vi "Add Custom Device Channel - Offline.vi"(4 "Property Values":variant[](array[variant]), 5 "Highlight? (F)":bool, 6 "Property names":string[](array[string]), 7 "GUID (Default Channel)":string="03D3BB99-1485-13A6-561D1F898F032919", 8 "error in (no error)":errorcluster, 9 "Channel":T2, 10 "Channel Name":string, 11 "Parent Ref in":T1 format="%.0x") -> (0 "error out":errorcluster, 1 "Channel Ref":T1 format="%.0x", 2 "Newly Created?":bool, 3 "Parent Ref out":T1 format="%.0x")   [LabVIEW 2017, in "Scan Engine Custom Device.lvlib"]
uses:
  Scan Engine Custom Device.lvlib
  <vilib>/NI Veristand/Custom Device API/Custom Device Item Ref.ctl
  <vilib>/NI Veristand/Custom Device API/Custom Device Channel.ctl
  <vilib>/NI Veristand/Custom Device API/Custom Device Channel Type.ctl
  NationalInstruments.VeriStand.SystemDefinitionAPI
  <vilib>/NI Veristand/Custom Device Offline API/Custom Device Offline API.lvlib
  <vilib>/NI Veristand/Custom Device API/Custom Device API.lvlib
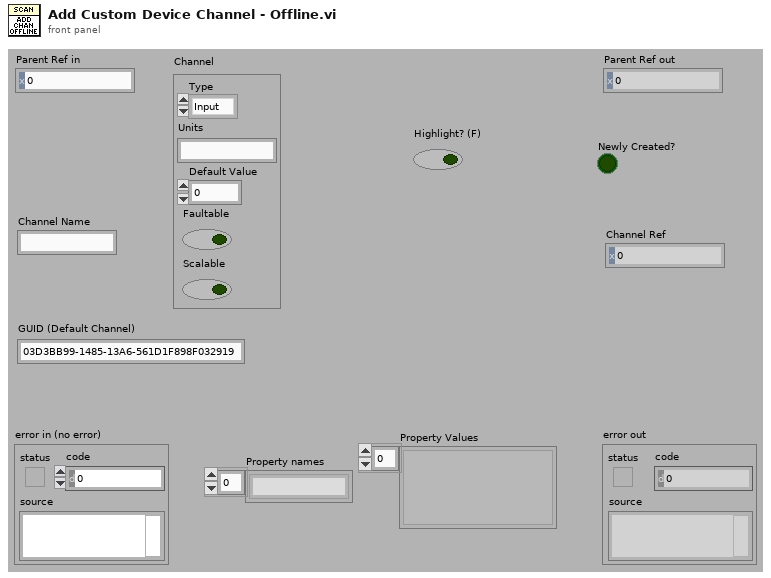
[diagram p1: front panel]
types:
  T1 = typedef "Custom Device API.lvlib/Custom Device Item Ref.ctl" = u64
  T2 = typedef "Custom Device API.lvlib/Custom Device Channel.ctl" = cluster{"Type":T3, "Units":string, "Default Value":dbl, "Faultable":bool, "Scalable":bool}
  T3 = typedef "Custom Device API.lvlib/Custom Device Channel Type.ctl" = enum16{"Input", "Output"}
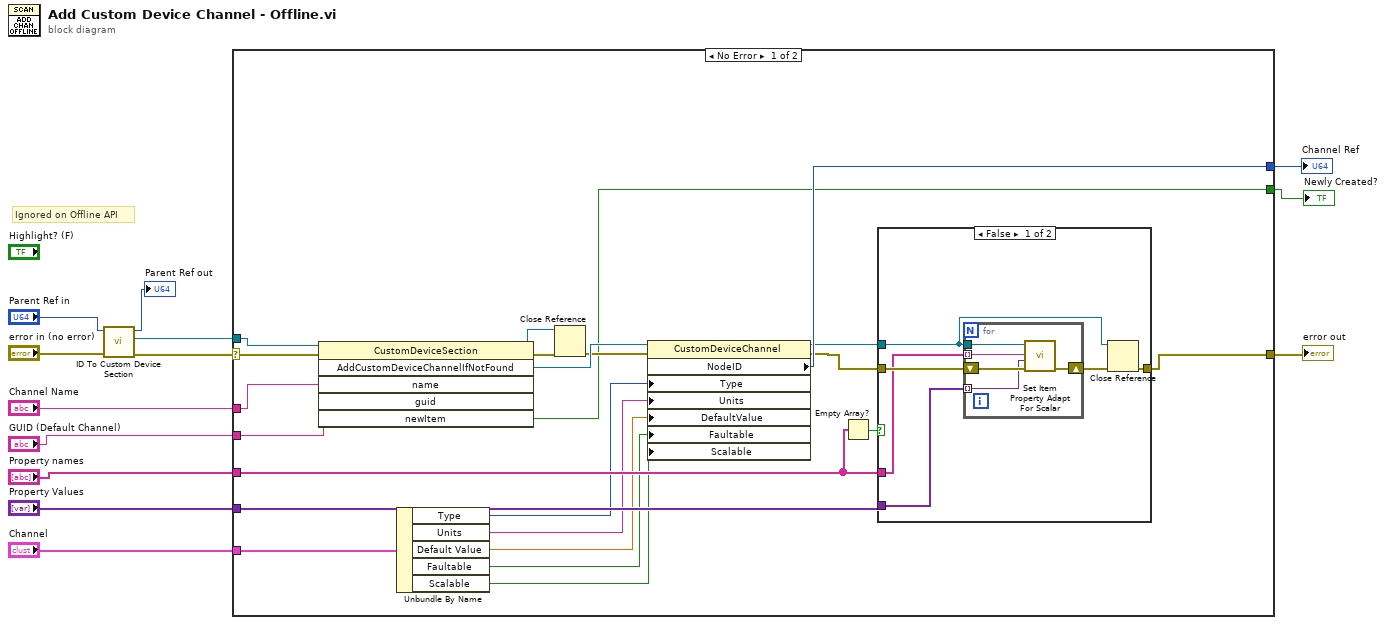
[diagram p0: block diagram]
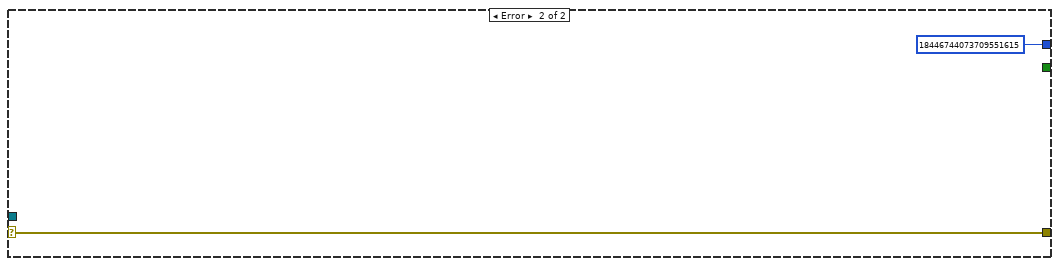
[diagram p3: hidden frame]
diagram:
  # "Ignored on Offline API"
  n1 = call <vilib>:"ID To Custom Device Section.vi"("error in (no error)"="error in (no error)", "ID in"="Parent Ref in") -> ("error out"=w13:errorcluster, "Section"=w12:refnum<k24>, "ID out"=→"Parent Ref out":u64)  [unwired: 7 in]
  n2 = case shown="No Error" w13 {
    selector: w13 -> [w34 w49]
    tunnel: [w32 w49] -> w2
    tunnel: w12 -> [w35 _]
    tunnel: "GUID (Default Channel)" -> [w33 _]
    tunnel: [w27 T1 18446744073709551615 ("Section Ptr")] -> w3
    tunnel: [w24 _] -> w4
    tunnel: "Property names" -> [w23 _]
    tunnel: "Property Values" -> [w22 _]
    tunnel: "Channel Name" -> [w21 _]
    tunnel: "Channel" -> [w20 _]
    frame No Error {
      n3 = invoke class="CustomDeviceSection" method="AddCustomDeviceChannelIfNotFound"(reference=w35, error in=w34, "name"=w21, "guid"=w33) -> (reference out=w30:refnum<k24>, error out=w31:errorcluster, "AddCustomDeviceChannelIfNotFound"=w29:refnum<k24>, "newItem"=w24:bool)  [unwired: 2 in, 2 out]
      n4 = Unbundle By Name(w20) -> ("Type"=w19:T3, "Units"=w18:string, "Default Value"=w17:dbl, "Faultable"=w16:bool, "Scalable"=w15:bool)
      n5 = Close Reference(reference=w30, error in (no error)=w31) -> (error out=w28:errorcluster)
      n6 = property class="CustomDeviceChannel"(reference=w29, error in=w28, "Type"=w19, "Units"=w18, "DefaultValue"=w17, "Faultable"=w16, "Scalable"=w15) -> (reference out=w25:refnum<k24>, error out=w26:errorcluster, "NodeID"=w27:u64)
      n7 = Empty Array?(array=w23) -> (empty?=w14:bool)
      n8 = case shown="False" w14 {
        tunnel: w25 -> [w37 _]
        tunnel: w26 -> [w41 w47]
        tunnel: w22 -> [w40 _]
        tunnel: w23 -> [w39 _]
        tunnel: [w36 w47] -> w32
        frame False {
          n9 = for {
            tunnel: w40 -> [w45] mode=indexing
            tunnel: w39 -> [w44] mode=indexing
            shift-right: [w42] -> w38
            shift-left: w41 -> [w46]
            tunnel: w37 -> [w43]
            n10 = call <vilib>:"Set Item Property Adapt For Scalar.vi"("error in (no error)"=w46, "Value"=w45, "Property Name"=w44, "CDBase"=w43) -> ("error out"=w42:errorcluster)  [unwired: 5 in, 2 out]
          }
          n11 = Close Reference(reference=w37, error in (no error)=w38) -> (error out=w36:errorcluster)
        }
        frame True {
        }
      }
    }
    frame Error {
    }
  }
  "error out" <- w2
  "Channel Ref" <- w3
  "Newly Created?" <- w4
